vi "Terminated.vi"(7 "Sender":refnum<class "Sender.lvclass">, 9 "Error":errorcluster, 10 "Actor":refnum<class "Actor.lvclass">, 11 "Base Actor in":refnum<class "Base Actor.lvclass">) -> (0 "Error out":errorcluster, 3 "Base Actor out":refnum<class "Base Actor.lvclass">)   [LabVIEW 2025, in "jettl.lvlib" / "Actor.lvlib" / "Base Actor.lvclass"]
uses:
  Base Actor.lvclass
  Base Actor.lvclass/Base Actor.ctl
  C:/git/jettl/src/jettl/jettl/Actor/Base Actor/Base Actor.lvclass
  C:/git/jettl/src/jettl/jettl/Actor/Actor/Actor.lvclass
  C:/git/jettl/src/jettl/jettl/Destroy Msg/Destroy/Destroy.lvclass
  C:/git/jettl/src/jettl/jettl/Terminated Msg/Terminated/Terminated.lvclass
  Actor.lvlib
  Destroy Msg/Destroy Msg.lvlib
  Actor/Actor.lvclass
  Attributes/Attributes/Attributes.lvclass
  Sender/Sender/Sender.lvclass
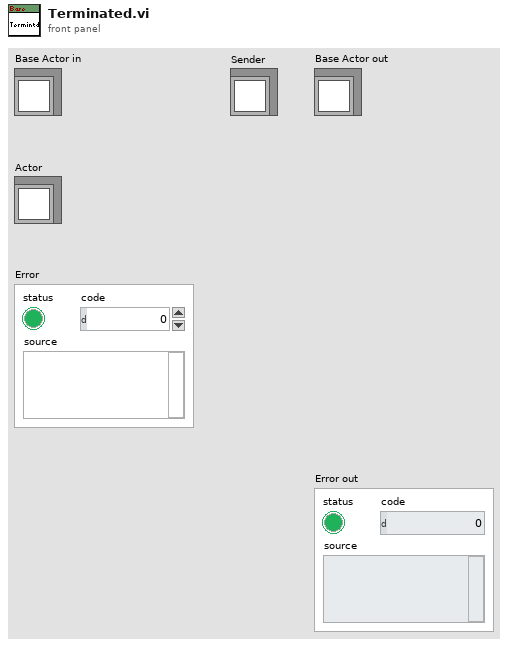
[diagram p1: front panel]
types:
  T1 = typedef "jettl.lvlib/Actor.lvlib/Relation.ctl" = enum16{"Self", "Creator", "Created"}
  T2 = typedef "jettl.lvlib/Actor.lvlib/Base Actor.lvclass/Created Attributes Map.ctl" = map{string, refnum<class "Attributes.lvclass">}
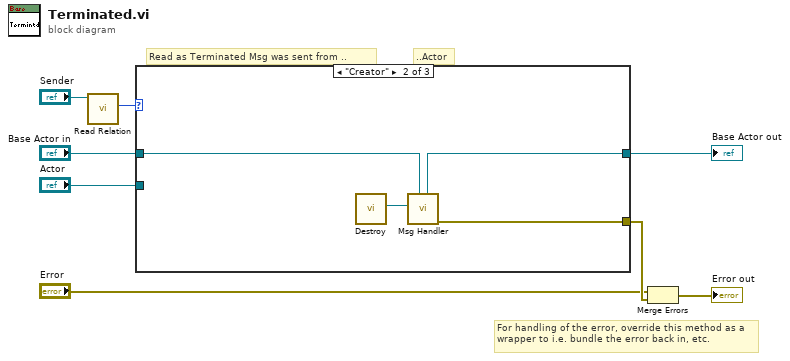
[diagram p0: block diagram]
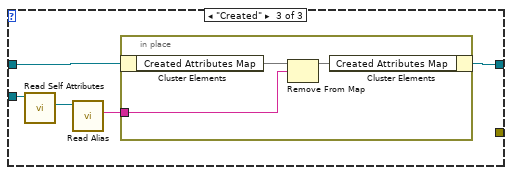
[diagram p3: hidden frame]
diagram:
  # "For handling of the error, override this method as a wrapper to i.e. bundle the error back in, etc."
  # "..Actor"
  # "Read as Terminated Msg was sent from .."
  n1 = call-dynamic "Read Relation.vi"("Sender in"="Sender") -> ("Relation"=w4:T1)  [unwired: 10 in]
  n2 = case shown="\"Creator\"" w4 {
    tunnel: "Base Actor in" -> [w9 w12 w17]
    tunnel: [w9 w11 w14] -> w8
    tunnel: "Actor" -> [_ _ w18]
    tunnel: [_ w13 _] -> w2
    frame "Self" {
      # "Case will not fundamentally execute"
    }
    frame "Creator" {
      n3 = call "Destroy.vi"() -> ("Msg"=w10:refnum<class "Msg.lvclass">)  [unwired: 11 in]
      n4 = call "Msg Handler.vi"("Actor in"=w12, "Msg"=w10) -> ("Error out"=w13:errorcluster, "Actor out"=w11:refnum<class "Base Actor.lvclass">)  [unwired: 8 in]
    }
    frame "Created" {
      n5 = call-dynamic "Read Self Attributes.vi"("Actor in"=w18) -> ("Self Attributes"=w16:refnum<class "Attributes.lvclass">)  [unwired: 10 in]
      n6 = call-dynamic "Read Alias.vi"("Attributes in"=w16) -> ("Alias"=w15:string)  [unwired: 10 in]
      n7 = in-place {
        in-place-border: w15 -> [w19]
        n8 = in-place-cluster #1(w17) -> ("Created Attributes Map"=w21:T2)
        n9 = Remove From Map(10:w19, 11:w21) -> (3:w20:T2)  [unwired: 2 out]
        n10 = in-place-cluster #1("Created Attributes Map"=w20) -> (w14:refnum<class "Base Actor.lvclass">)
      }
    }
  }
  "Base Actor out" <- w8
  n11 = Merge Errors("Error", w2) -> (→"Error out":errorcluster)
